vi "KI6221.vi"() -> ()   [LabVIEW 2019] (continued)
  in  "RUN ARB .H":string="The RUN ARB code initiates an ARB waveform. When you see something like \"<PMARK>\" this is a variable. These are replaced with values before being sent to the instrument. Many are self explanatory. DURATION is in seconds and FREQUENCY is in Hz. When you see WAIT1500 that indicates a delay in ms. (i.e. a 1500 ms delay between these commands). When you see ENTER256 this indicates you need to read data from the box. The number is the recommended number of bytes to read. "
  in  "UPLOAD ARB .H":string="The UPLOAD ARB code aborts any other sweep running, turns off the output, then loads an ARB wave. When you see something like \"<PULSELEVEL>\" this is a variable. These are replaced with values before being sent to the instrument. Many are self explanatory. The command sour:wave:arb1:data <WAVEFORM> will upload the waveform to the instrument. The variable needs to be replaced with a sequence of numbers between -1 and 1 separated by commas. I.E. \"1,.5,0,-.5,-1\". The command can only take data about 1000 bytes of ASCII or smaller at a time, so if your waveform is larger than that separate them and use the :sour:wave:arb:append <WAVEFORM> command to add more points. When you see WAIT1500 that indicates a delay in ms. (i.e. a 1500 ms delay between these commands). When you see ENTER256 this indicates you need to read data from the box. The number is the recommended number of bytes to read. "
  in  "RUN PULSE .H":string="The RUN PULSE code aborts any other sweep running, resets the instrument, then sets up a PULSE series. When you see something like \"<PULSELEVEL>\" this is a variable. These are replaced with values before being sent to the instrument. Many are self explanatory. We set the <PULSESWEEPSTATE> to a binary value 1 or 0 depending on whether we want to sweep or repeat pulses. The strings ON and OFF will also work. The <PULSESWEEPINT> variable is used to set the sweep delay. We find that the most repeatable pulses in sweep mode come when you set the delay to 6 ms less than the time that equals the number of NPLCs requested. So the formula for <PULSESWEEPINT> is (NPLC*1/Power_Line_Freq - 6)/1000. The :syst:comm:serial:send command allows communication to the Model 2182 over RS-232. When you see WAIT1500 that indicates a delay in ms. (i.e. a 1500 ms delay between these commands). You may find you have to place additional delays especially when using the RS-232 pass through commands. When you see ENTER256 this indicates you need to read data from the box. The number is the recommended number of bytes to read."
  in  "RUN DC .H":string="The RUN DIFF COND code aborts any other sweep running, resets the instrument, then sets up a DIFF COND sweep. When you see something like \"<DCONSTOP>\" this is a variable. These are replaced with values before being sent to the instrument. Many are self explanatory. We set the DCONSTEP value to (STOP-START)/((NUMPOINTS-1)*FILTERCOUNT) and the DCONDELTA (amplitude of the square wave superimposed on the sweep) is set to STEPSIZE*FILTERCOUNT. The :syst:comm:serial:send command allows communication to the Model 2182 over RS-232. When you see WAIT1500 that indicates a delay in ms. (i.e. a 1500 ms delay between these commands). When you see ENTER256 this indicates you need to read data from the box. The number is the recommended number of bytes to read."
  in  "RUN DELTA .H":string="The RUN DELTA Code aborts any other sweep running, resets the instrument, then sets up a DELTA sweep. When you see something like \"<DELTAHIGH>\" this is a variable. These are replaced with values before being sent to the instrument. Many are self explanatory. The var <DELTACURRRANGE> is the current range and it can be replaced with a numeric string like \" .002\" (2 mA range) or with a string like \":auto on\" which turns auto range on. All other variables will have a space before them. The :syst:comm:serial:send command allows communication to the Model 2182 over RS-232. When you see WAIT1500 that indicates a delay in ms. (i.e. a 1500 ms delay between these commands). When you see ENTER256 this indicates you need to read data from the box. The number is the recommended number of bytes to read."
  out "error out 25":errorcluster
  out "error out 24":errorcluster
  out "error out 23":errorcluster
  out "DELTA SCPI ERROR 2":errorcluster
  out "error out 17":errorcluster
  out "error out 16":errorcluster
  out "Knob Last":i16
  out "Control watch":bool=TRUE
  out "error out 21":errorcluster
  out "error 27":errorcluster
  out "error out 15":errorcluster
  out "SETUP YET?":i32
  out "error out 14":errorcluster
  out "error out 13":errorcluster
  out "VALID SETUP":bool
  out "error out 12":errorcluster
  out "step VISA":refnum<visa-resource-name>="GPIB0::24::INSTR"
  out "6220 VISA":refnum<visa-resource-name>="TCPIP0::10.40.27.160::1394::SOCKET"
  out "GPIB Array":string[](array[string])=["*idn?\nENTER1024", ":SYST:COMM:SERIal:SEND \"*idn?\"\nWAIT1000\n:SYST:COMM:SERIal:enter?\nWAIT1000\nENTER2000", ":disp:data?\nENTER256\n:disp:wind2:data?\nENTER256\n:outp:stat?\nENTER256\n:disp:attr?\nENTER256\n:disp:wind2:attr?\nENTER256", ":syst:key <KEYPRESS>", ":trac:poin:act?\nENTER256", ":sour:wave:arb:append <APPEND>\nWAIT30", "*rst", ":disp:data?\nENTER256\n:disp:wind2:data?\nENTER256\n:outp:stat?\nENTER256\n:disp:attr?\nENTER256\n:disp:wind2:attr?\nENTER256", "sour:swe:abort\nWAIT500\nSOUR:WAVE:ABOR\nWAIT500\noutp:stat off\nsour:wave:ampl <AMPLITUDE>\nsour:wave:offs <OFFSET>\nsour:wave:arb:data <WAVEFORM>\nWAIT300\t", "SOUR:WAVE:ABOR\nWAIT300\n:outp:stat off\n<SETUPSTRING>\nWAIT500\nsour:wave:arb:copy 1\nWAIT3000\nsour:wave:func ARB0\nWAIT1000\nsour:wave:rang best\nsour:wave:pmar:stat <PMARK_ENABLE>\nsour:wave:pmar <PMARK>\nsour:wave:pmar:olin <TRIGGERLINE>\nsour:wave:freq <FREQUENCY>\nsour:wave:dur:time <DURATION>\n:sour:curr:comp <ARBCOMP>\nsour:wave:arm\nWAIT2000\n:outp:stat on\nWAIT500\nsour:wave:init", "SOUR:WAVE:ABOR\noutp:stat off", "sour:wave:arb:poin?\nENTER256", ":sour:delta:nvpr?\nENTER256", ":sour:dcon:nvpr?\nENTER256", ":SYST:COMM:SERIal:SEND \"*rst\"\nWAIT1500\n:sour:pdel:nvpr?\nENTER256", "SOUR:WAVE:ABOR\noutp:stat off\n*rst", ":sour:swe:abort\n*rst\n<SETUPSTRING>\nWAIT500\n:form:elem READ,TST,RNUM,AVOL\n:sour:delt:high <DELTAHIGH>\n:sour:delt:low <DELTALOW>\n:sour:delt:count <DELTANUMCYCLE>\n:sour:delt:delay <DELTADELAY>\n:sour:curr:filt:stat <DELTADAMPING>\n:sour:curr:comp <DELTACOMP>\n:sour:curr:rang<DELTACURRRANGE>\n:SYST:COMM:SERIal:SEND \"*rst\"\nWAIT400\n:SYST:COMM:SERIal:SEND \":sens:volt:nplc <DELTANPLC>\"\nWAIT1500\n:SYST:COMM:SERIal:SEND \":sens:volt:rang <DELTAVOLTRANGE>\"\n:sens:aver:wind 0\n:sens:aver:stat <DELTAFILTERSTATE>\n:sens:aver:coun <DELTAFILTERCOUNT>\n:sens:aver:tcon <DELTAFILTERTYPE>\n:sour:delt:arm\nWAIT1000\n:init:imm", ":sour:swe:abort\n:outp:stat off", ":sour:swe:abort\n:outp:stat off", ":trac:data:sel? <DATASTART>,<DATACOUNT>\nENTER40000", ":sour:swe:abort\nWAIT3000\n*rst\n<SETUPSTRING>\nWAIT500\n:form:elem READ,TST,RNUM,SOUR\n:sour:pdel:high <PULSEHIGH>\n:sour:pdel:low <PULSEOFF>\n:sour:pdel:count <PULSECOUNT>\n:sour:pdel:rang best\n:sour:swe:rang best\n:sour:pdel:width <PULSEWIDTH>\n:sour:pdel:sdel <PULSEDELAY>\n:sour:pdel:swe <PULSESWEEPSTATE>\n:sour:pdel:int <PULSEINTERVAL>\n:sour:curr:comp <PULSECOMP>\n:sour:swe:spac <PULSESWEEPSPACING>\n:sour:curr:start <PULSESWEEPSTART>\n:sour:curr:stop <PULSESWEEPSTOP>\n:sour:curr:step <PULSESWEEPSTEP>\n:SYST:COMM:SERIal:SEND \":sens:volt:rang <PULSEVOLTRANGE>\"\n:sens:aver:wind 0\n:sens:aver:stat <PULSEFILTERSTATE>\n:sens:aver:coun <PULSEFILTERCOUNT>\n:sens:aver:tcon <PULSEFILTERTYPE>\n:sour:pdel:arm\nWAIT3000\n:init:imm", ":sour:swe:abort\n:outp:stat off", ":sour:swe:abort", ":trac:data:sel? 0,<DATACOUNT>\nENTER4000000", ":sour:swe:abort\n*rst\n<SETUPSTRING>\nWAIT500\n:form:elem READ,TST,RNUM,SOUR,AVOL\n:sour:dcon:start <DCONSTART>\n:sour:dcon:stop <DCONSTOP>\n:sour:dcon:step <DCONSTEP>\n:sour:dcon:del <DCONDELAY>\n:sour:dcon:delt <DCONDELTA>\n:sour:curr:comp <DCONCOMP>\n:sour:curr:filt:stat <DCONDAMPING>\n:SYST:COMM:SERIal:SEND \":sens:volt:rang <DCONVOLTRANGE>\"\nWAIT700\n:SYST:COMM:SERIal:SEND \":sens:volt:nplc <DCONNPLC>\"\nWAIT500\n:sens:aver:wind 0\n:sens:aver:stat <DCONFILTERSTATE>\n:sens:aver:coun <DCONFILTERCOUNT>\n:sens:aver:tcon REPEAT\nWAIT2000\n:sour:dcon:arm\nWAIT3000\n:init:imm", ":sour:swe:abort\n:outp:stat off", ":sour:swe:abort", ":sour:swe:abort\nWAIT2000\n:outp:stat off\n*rst\nWAIT1000\n:sour:curr:comp <AUTOCOMP>\n:sour:curr:filt:stat <DCONDAMPING>\n:SYST:COMM:SERIal:SEND \"*rst\"\nWAIT800\n:SYST:COMM:SERIal:SEND \":sens:volt:rang <DCONVOLTRANGE>\"\nWAIT200\n:SYST:COMM:SERIal:SEND \":sens:volt:rang:auto on\"\nWAIT200\n:SYST:COMM:SERIal:SEND \":sens:volt:nplc <DCONNPLC>\"\nWAIT200", ":sour:curr:rang <STARTLEVEL>\n:sour:curr:lev <STARTLEVEL>\n:outp:stat on\nWAIT200\n:sour:curr:rang <CURRENTLEVEL>\n:sour:curr:lev <CURRENTLEVEL>\nWAIT500\n:SYST:COMM:SERIal:SEND \":read?\"\nWAIT1000\n:SYST:COMM:SERIal:enter?\nENTER512", ":sour:curr:rang <SOURCE>\n:sour:curr:lev <SOURCE>\n:sour:curr:comp <COMPLIANCE>\n:outp:stat <OUTPUT>", ":sour:swe:abort\n*rst\n<SETUPSTRING>\nWAIT1000\n:sour:swe:spac <SPACING>\n:sour:swe:poin <POINTS>\n:sour:swe:rang best\n:sour:swe:coun 1\n:sour:swe:cab off\n:sour:curr:start <STARTLEVEL>\n:sour:curr:stop <STOPLEVEL>\n:sour:curr:comp <COMPLIANCE>\n:sour:del <DELAY>\nWAIT1000\n:sour:swe:arm\nWAIT3000\n:init:imm", ":sour:swe:abort\n:outp:stat off", "#33 basic AC Source STOP%", "#34 wAIT%\nWAIT2000", "WAIT2000", ":sour:swe:abort\n*rst\n:SYST:COMM:SERIal:SEND \"*rst\"\n<SETUPSTRING>\nWAIT1000\n:sour:swe:spac <SPACING>\n:sour:swe:poin <POINTS>\n:sour:swe:rang best\n:sour:swe:coun 1\n:sour:swe:cab off\n:sour:curr:start <STARTLEVEL>\n:sour:curr:stop <STOPLEVEL>\n:sour:curr:comp <COMPLIANCE>\n:sour:del <DELAY>\n:trig:sour tlink\n:trig:dir sour\n:trig:olin 2\n:trig:ilin 1\n:trig:outp del\n:SYST:COMM:SERIal:SEND \":sens:volt:rang <VOLTRANGE>\"\nWAIT400\n:SYST:COMM:SERIal:SEND \":sens:volt:nplc <NPLC>\"\nWAIT400\n:SYST:COMM:SERIal:SEND \":trac:cle\"\nWAIT200\n:SYST:COMM:SERIal:SEND \":trac:feed sens\"\nWAIT200\n:SYST:COMM:SERIal:SEND \":trac:poin <POINTS>\"\nWAIT200\n:SYST:COMM:SERIal:SEND \":trig:sour ext\"\nWAIT200\n:SYST:COMM:SERIal:SEND \":trig:coun <POINTS>\"\nWAIT200\n:SYST:COMM:SERIal:SEND \":trac:feed:control next\"\nWAIT500\n:sour:swe:arm\nWAIT1000\n:init:imm\n:SYST:COMM:SERIal:SEND \"init\"", ":sour:swe:abort\n:outp:stat off\n*rst\n:SYST:COMM:SERIal:SEND \"*rst\"\n:trig:olin 4", "*idn?\nENTER1024\n:sour:swe:abort\n*rst\n<SETUPSTRING>\nWAIT1000", ":SYST:COMM:SERIal:SEND \":trac:data?\"\nWAIT200\n:SYST:COMM:SERIal:enter?\nENTER40000", ":sour:wave:abor\nWAIT300\n:outp:stat off\n*rst\nWAIT2000\n<SETUPSTRING>\n:sour:curr:comp <ACCOMPLIANCE>\n:sour:wave:func ramp\n:sour:wave:rang best\n:sour:wave:dcycle <RAMPDUTYCYCLE>\n:sour:wave:ampl <RAMPAMPLITUDE>\n:sour:wave:freq <FREQUENCY>\n:sour:wave:offset <RAMPOFFSET>\n:sour:wave:dur:time inf\n:sour:wave:arm\nWAIT3000\n:sour:wave:init", ":sour:wave:abor\nWAIT300\n:outp:stat off\n*rst\nWAIT2000\n<SETUPSTRING>\nWAIT500\n:sour:curr:comp <ACCOMPLIANCE>\n:sour:wave:func square\n:sour:wave:dcycle <SQUAREDUTYCYCLE>\n:sour:wave:ampl <SQUAREAMPLITUDE>\n:sour:wave:freq <FREQUENCY>\n:sour:wave:offset <SQUAREOFFSET>\n:sour:wave:rang best\n:sour:wave:dur:time inf\n:sour:wave:arm\nWAIT3000\n:sour:wave:init", ":sour:wave:abor\nWAIT300\n:outp:stat off\n*rst\nWAIT2000\n<SETUPSTRING>\nWAIT500\n:sour:curr:comp <ACCOMPLIANCE>\n:sour:wave:func sin\n:sour:wave:ampl <SINEAMPLITUDE>\t\t\n:sour:wave:freq <FREQUENCY>\n:sour:wave:offset <SINEOFFSET>\n:sour:wave:rang best\n:sour:wave:dur:time inf\n:sour:wave:arm\nWAIT3000\n:sour:wave:init", ""]
  out "error out 10":errorcluster
  out "error out 7":errorcluster
  out "triggerline":i16=1 min=0 max=5
  out "Phase Value":dbl min=0.0 max=360.0
  out "phase enable":bool
  out "error out 5":errorcluster
  out "selection":dbl[](array[numeric])=[2.01, 2.01, 2.01, 2.01, 2.01, 1.99, 1.99, 1.99, 1.99, 1.99, 2.01, 2.01, 2.01, 2.01, 2.01, 1.99, 1.99, 1.99, 1.99, 1.99, 2.01, 2.01, 2.01, 2.01, 2.01, 1.99, 1.99, 1.99, 1.99, 1.99, 2.01, 2.01, 2.01, 2.01, 2.01, 1.99, 1.99, 1.99, 1.99, 1.99, 2.01, 2.01, 2.01, 2.01, 2.01, 1.99, 1.99, 1.99, 1.99, 1.99, 2.01, 2.01, 2.01, 2.01, 2.01, 1.99, 1.99, 1.99, 1.99, 1.99, 2.01, 2.01, 2.01, 2.01, 2.01, 1.99, 1.99, 1.99, 1.99, 1.99, 2.01, 2.01, 2.01, 2.01, 2.01, 1.99, 1.99, 1.99, 1.99, 1.99, 2.01, 2.01, 2.01, 2.01, 2.01, 1.99, 1.99, 1.99, 1.99, 1.99, 2.01, 2.01, 2.01, 2.01, 2.01, 1.99, 1.99, 1.99, 1.99, 1.99]
  out "Pad Last":i32=-2
  out "Graph Last":i32=-2
  in  "waveform holder":dbl[](array[numeric])
  out "empty":dbl[](array[numeric])
  out "Complete Array Cnt":i32[](array[numeric])
  out "ScratchPad Array Cnt":i32[](array[numeric])=[100, 100, 100, 100, 0]
  out "Default path":path=path "C:/6220software/data"
  out "error out 6":errorcluster
  out "Complete Array":dbl[][](array[numeric])
  out "ScratchPad Array":dbl[][](array[numeric])
  in  "mail server":string
  in  "attachments":T6(array[cluster])=[{"path"=path "C:/6220software/data/DefaultTestFile.cfg", "data"="", "binary"=FALSE, "MIME content-type \n(application/octet-stream)"=""}, {"path"=path "C:/6220software/data/DefaultTestFile_dcdata.cfg", "data"="", "binary"=FALSE, "MIME content-type \n(application/octet-stream)"=""}, {"path"=path "C:/6220software/data/DefaultTestFile_pulsedata.cfg", "data"="", "binary"=FALSE, "MIME content-type \n(application/octet-stream)"=""}, {"path"=path "C:/6220software/data/DefaultTestFile_deltadata.cfg", "data"="", "binary"=FALSE, "MIME content-type \n(application/octet-stream)"=""}]
  out "error out 4":errorcluster
  out "Y AXIS LAST -PULSE":i32=-1
  in  "Y AXIS LAST -DC":i32=-1
  out "Y AXIS LAST -DELTA":i32
  out "X AXIS LAST -PULSE":i32
  in  "X AXIS LAST -DC":i32
  out "X AXIS LAST -DELTA":i32
  out "DELTA SCPI ERROR":errorcluster
  out "Settings cluster":T7={"Boolean"=TRUE, "Numeric"=5.0, "y"=timestamp(3168632206.8599997 s since 1904-01-01), "version"="2.6", "y 2"=timestamp(3168632206.8599997 s since 1904-01-01)}
  out "FIRST OPEN":bool
  out "Last setup Cluster":T8={"Numeric"=2, "Numeric 2"=3, "Numeric 3"=1, "Numeric 4"=10, "Numeric 5"=40, "Numeric 6"=27, "Numeric 7"=160, "Numeric 8"=0, "Numeric 9"=16, "Numeric 10"=0, "Numeric 11"=1, "Numeric 12"=0, "Numeric 13"=0, "Boolean"=FALSE, "Numeric 14"=0, "Numeric 15"=0}
  out "error out 2":errorcluster
  in  "Default Cluster":T8={"Numeric"=2, "Numeric 2"=3, "Numeric 3"=1, "Numeric 4"=10, "Numeric 5"=40, "Numeric 6"=27, "Numeric 7"=160, "Numeric 8"=0, "Numeric 9"=16, "Numeric 10"=0, "Numeric 11"=1, "Numeric 12"=0, "Numeric 13"=0, "Boolean"=FALSE, "Numeric 14"=0, "Numeric 15"=0}
  out "MASTER DRIVER Array":T9(array[cluster])=[{"Numeric"=24, "String"="2400", "String 2"="*IDN?", "String 3"="2400", "String 4"="*rst\n:sour:func volt\n:outp:stat on", "String 5"=":sour:volt:lev <LEVEL>", "String 6"=":outp:stat off", "Numeric 2"=20}, {"Numeric"=20, "String"="Window Pop-up", "String 2"="", "String 3"="", "String 4"="THIS IS A SPECIAL SETUP FUNCTION THAT CREATES A POP-UP WINDOW SO YOU CAN SET SOME MANUAL EXTERNAL DEVICE TO THE APPROPRIATE STEP VALUES.\nDO NOT EDIT THIS SETUP OR CHANGE THE INSTRUMENT NAME.", "String 5"="", "String 6"="", "Numeric 2"=20}, {"Numeric"=20, "String"="NEW...", "String 2"="", "String 3"="", "String 4"="", "String 5"="", "String 6"="", "Numeric 2"=20}]
  out "STEP EDIT VAR":bool
  out "output cluster":T10={"Value"=0.0004, "Value"=50, "Value"=1, "Value"=FALSE, "Value"=-0.0004, "Value"=1000, "Value"=0, "Value"=1.0, "Value"=0.01, "Value"=FALSE, "Value"=1.0, "Value"=10.0, "Value"=0, "Value"=0.0, "Value"=-0.001, "Value"=101, "Value"=0.0, "Value"=0.001, "Value"=2, "Value"=101, "Value"=1, "Value"=0, "Value"=2.0, "Value"=0.0, "Value"=1, "Value"=FALSE, "Value"=1.0, "Value"=100, "Value"=2, "Value"=2, "Value"=0.01, "Value"=0.0, "Value"=0, "Value"=10.0, "Value"=1.0, "Value"=100.0, "Value"=0.1, "Value"=0, "Value"=10000.0, "Value"=100, "complete number of cycles"=10.0, "Value"=20, "Value"=0.016, "Value"=0.05, "Value"=0.01, "Value"=0.01, "Value"=0.0, "Value"=0, "Value"=0.05, "Value"=100.0, "Value"=10.0, "Value"=0, "Value"=1, "Value"=FALSE, "Value"=40, "Value"=3, "Value"=0, "Value"=FALSE, "Value"=1, "Value"=10, "Value"=0, "Value"=0, "Value"=1, "Value"=27, "Value"=TRUE, "Value"=2, "Value"=160, "Value"=16, "Value"=TRUE, "Value"=0, "result string"="2400", "result string"="*rst\n:sour:func volt\n:outp:stat on", "result string"=":outp:stat off", "result string"=":sour:volt:lev <LEVEL>", "result string"="*IDN?", "result string"="2400", "Value"=20, "Value"=24, "Value"=FALSE, "String"="Enter details to remember about this test here. It will be saved with your test file.", "PULSE - SWEEP #STEPS"=101, "Sawtooth NUM CYCLES"=5.0, "Sawtooth Offset (Amps) 2"=0.01, "Duty Cycle (%) 2"=50.0, "Start Phase \n(Degrees) 2"=0.0, "SQUARE Number of Points per cycle 2"=10, "SQUARE Number of Cycles 2"=10.0, "SQUARE Amplitude (Amps) 2"=0.01, "SQUARE Offset (Amps) 2"=0.0, "SQUARE Duty Cycle (%) 3"=50.0, "SQUARE Start Phase \n(Degrees) 3"=0.0, "SQUARE Rise/Fall in points 2"=1, "SINE Number of Points per cycle 2"=100, "SINE Number of Cycles 2"=1.0, "SINE Amplitude (Amps) 2"=0.05000000000000075, "SINE Offset (Amps) 2"=0.0, "SINE Start Phase \n(Degrees) 3"=0.0, "NOISE Number of Points per cycle 2"=100, "NOISE Number of Cycles 2"=1.0, "NOISE Standard Deviation 2"=0.01, "NOISE Offset (Amps) 2"=0.0, "Analog filter - \nTau in # points 2"=1.0, "ScratchPad Array 2"=array4x66001[264004 elements], "ScratchPad Array Cnt 2"=[100, 100, 100, 100, 0], "Item Names"=["RAMP0", "SQUARE0", "SINE0", "NOISE0"], "ADD 5"=[2], "Complete Array 2"=[], "Complete Array Cnt 2"=[0], "Item Names 5"=[], "ADD 7"=[0], "waveform holder 2"=[], "ADD 6"=[1], "ADD 8"=[1], "ADD 9"=[1], "Trace offset (% Pk-Pk): 2"=0.0, "phase enable 2"=FALSE, "Phase Value 2"=0.0, "triggerline 2"=1, "Pulse Off Level (Amps) 2"=0.0, "ARB VOLT COMP"=10.0, "nV CAP"=0, "Pulse Filter"=0, "Pulse FIlter Count"=2, "Setup String"=":SYST:COMM:SERIal:SEND \"SYST:FFIL ON\"\r\n:OUTP:ISH OLOW\r\n:outp:lte OFF", "DCON filter state"=0, "Source Level (Amps) 3"=0.0, "Current Source \nVoltage Compliance (V) 4"=10.01, "Start Current (Amps) 3"=0.001, "Stop Current (Amps) 3"=0.005, "Number of sweep points 3"=50, "Sweep Type 3"=0, "Current Source \nVoltage Compliance (V) 5"=10.0, "Delay (settle time in sec) 3"=0.01, "enable measure 3"=TRUE, "Voltage Measure Range 3"=0.1, "Measurement Integration \n(NPLCs) 3"=1.0, "Waveform Type  3"=1, "I Sweep V Measure Data 3"=[], "Ramp from: (Amps) 3"=0.0, "Ramp to: (Amps) 3"=0.0, "Duty Cycle (%) 4"=50.0, "Amplitude (Amps) 4"=0.105, "Offset (Amps) 4"=0.0, "Duty Cycle (%) 5"=50.0, "Amplitude (Amps) 5"=2e-12, "Offset (Amps) 5"=0.01, "Signal Repetition \nFrequency (Hz) 3"=10.0, " Voltage\n Compliance3"=10.0, "Number of Zero Measurements 2"=0} {"Number of Zero Measurements 2" min=0 max=2 step=1; "Voltage\n Compliance3" min=0.1 max=105.0 step=0.01 format="%#_3f"; "Signal Repetition \nFrequency (Hz) 3" min=0.0001 max=100000.0 format="%.4f"; "Offset (Amps) 5" min=-0.105 max=0.105 step=1e-12 format="%^#.6g"; "Amplitude (Amps) 5" min=2e-12 max=0.105 step=1e-12 format="%^#_6g"; "Duty Cycle (%) 5" min=0.0 max=100.0 format="%#.2f"; "Offset (Amps) 4" min=-0.105 max=0.105 step=1e-12 format="%^#_6g"; "Amplitude (Amps) 4" min=0.0 max=0.105 step=1e-12 format="%^#.6g"; "Duty Cycle (%) 4" min=0.0 max=100.0 format="%#.2f"; "Ramp to: (Amps) 3" min=-0.105 max=0.105 step=1e-12 format="%^#_6g"; "Ramp from: (Amps) 3" min=-0.105 max=0.105 step=1e-12 format="%^#.6g"; "Waveform Type  3" items=["RAMP", "SQUARE", "SINE"]; "Measurement Integration \n(NPLCs) 3" items=["0.01"=0.01, "0.1"=0.1, "1"=1.0, "10"=10.0]; "Voltage Measure Range 3" items=["10 mV"=0.01, "100 mV"=0.1, "1 V"=1.0, "10 V"=10.0, "100 V"=100.0]; "Delay (settle time in sec) 3" min=0.001 max=9999000.0 format="%^#_6g"; "Current Source \nVoltage Compliance (V) 5" min=0.1 max=105.0 step=0.01 format="%^#_6g"; "Sweep Type 3" items=["Linear ", "Logarithmic"]; "Number of sweep points 3" min=2 max=65536; "Stop Current (Amps) 3" min=-0.105 max=0.105 format="%^#_6g"; "Start Current (Amps) 3" min=-0.105 max=0.105 format="%^#_6g"; "Current Source \nVoltage Compliance (V) 4" min=0.1 max=105.0 step=0.01 format="%^#_6g"; "Source Level (Amps) 3" min=-0.105 max=0.105 step=1e-12 format="%^#_9e"; "Pulse Off Level (Amps) 2" min=-0.1 max=0.1 format="%^#_3e"; "triggerline 2" min=0 max=5; "Phase Value 2" min=0.0 max=360.0; "Analog filter - \nTau in # points 2" min=1.0; "NOISE Offset (Amps) 2" min=-10.0 max=10.0 format="%^#_6e"; "NOISE Standard Deviation 2" min=0.0 max=1.0 format="%^#_6e"; "NOISE Number of Cycles 2" min=1.0 max=65536.0; "NOISE Number of Points per cycle 2" min=1 max=65536 format="%#.0f"; "SINE Start Phase \n(Degrees) 3" min=0.0 max=360.0 format="%#.3f"; "SINE Offset (Amps) 2" min=-10.0 max=10.0 step=1e-17 format="%#.2f"; "SINE Amplitude (Amps) 2" min=-10.0 max=10.0 step=1e-12 format="%^#_6e"; "SINE Number of Cycles 2" min=1.0 max=65536.0; "SINE Number of Points per cycle 2" min=1 max=65536 format="%#.0f"; "SQUARE Rise/Fall in points 2" min=1; "SQUARE Start Phase \n(Degrees) 3" min=0.0 max=360.0 format="%#.3f"; "SQUARE Duty Cycle (%) 3" min=0.0 max=100.0 format="%#.2f"; "SQUARE Offset (Amps) 2" min=-10.0 max=10.0 format="%^#_6e"; "SQUARE Amplitude (Amps) 2" min=-10.0 max=10.0 format="%^#.6e"; "SQUARE Number of Cycles 2" min=1.0; "SQUARE Number of Points per cycle 2" min=1; "Start Phase \n(Degrees) 2" min=0.0 max=360.0 format="%#.3f"; "Duty Cycle (%) 2" min=0.0 max=100.0 format="%#.2f"; "Sawtooth Offset (Amps) 2" min=-10.0 max=10.0 format="%^#_6e"; "Sawtooth NUM CYCLES" min=1.0}
  out "SAVE NOW":bool
  out "EXIT NOW":bool
  # "Model 6220/6221 Current Source Example Software"
  # "Instrument Communication"
  # "Last Saved settings open on startup..."
  # "Instrument Selection"
  # "Source Connection"
  # "Measure Connection"
  # "Communication Configuration"
  # "Earth Connection"
  # "Input Capacitance"
  # "Step-By-Step Instrument Connection Tutorial"
  # "Connect communication cables as shown:"
  # "Connect the current source to the DUT as shown:"
  # "Connect the nanovoltmeter to the DUT as shown:"
  # "Select problems to view best shielding configuration:"
  # "Data Sheet"
  # "Data Sheet"
  # "Horizontal and Vertical Axis are controlled from 2-D Graph Tab"
  # "Data Sheet"
  # "Z data controlled by step source values:"
  # "For one sweep, set # of steps to 1 and set the Start Level."
  # "Data Sheet"
  # "Waveforms     ----------->               ScratchPad                 ------>                Complete waveform settings"
  # "Browse to a file containing your points. File should be\na text file with CRLFs between each point. This is the\ntype of waveform where you can customize a wave\nin a spreadsheet editor or other tool. Simply, create a\nsingle column of data points in column A on a blank\nsheet and select to save the sheet as a text file. This\nshould work by default, but it can be checked by \nopening with Notepad. Data should appear as a \ncolumn of text with carriage returns after each point."
  # "Select the waves you wish to combine in a calculation\nor check the box next to Constant and use the left \nselection and constant in scalar math.\nThen click CREATE."
  # "Select a waveform from the scratchpad to apply an\nanalog filter. Then click CREATE."
  # "6220 Virtual Instrument Front Panel"
  # "First, click Take Control of Instrument. Then use buttons and knobs below as you would from the instrument front panel. \nConnection uses settings on Instrument Communication Panel."
  # "Go Online..."
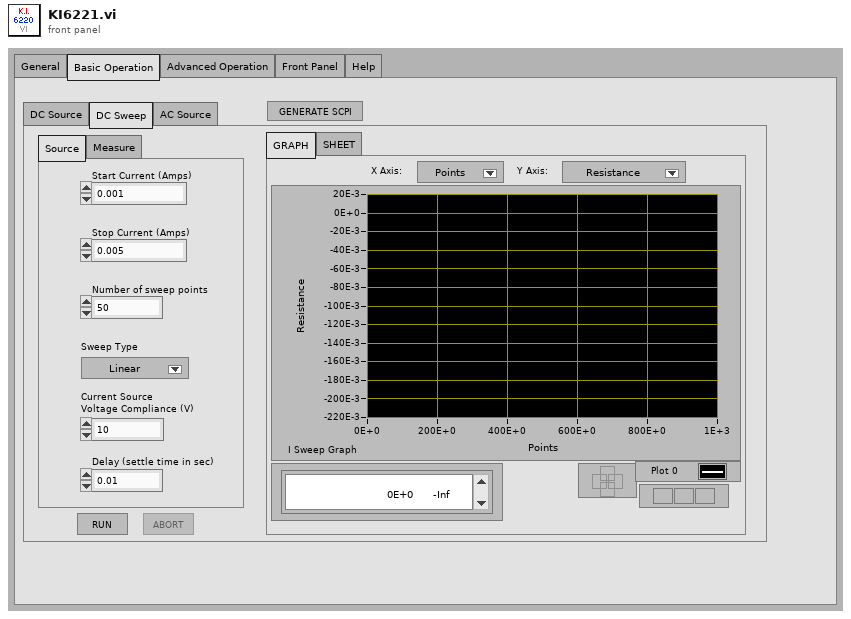
[diagram p1: front panel]
types:
  T1 = enum32{"General", "Basic Operation", "Advanced Operation", "Front Panel", "Help"}
  T2 = enum32{"STARTUP", "CONN CONFIG", "CONN GUIDE", "STEP CONFIG"}
  T3 = enum32{"step 1", "step 2", "step 3", "step 4", "final"}
  T4 = enum32{"Delta Mode Measurements", "Differential Conductance Measurements", "Pulsed IV Measurements", "ARB Waveform Generator", "6220 Virtual Front Panel", "Instrument Communication"}
  T5 = enum32{"RAMP", "SQUARE", "SINE", "NOISE", "CUSTOM", "CALCULATED", "FILTER"}
  T6 = cluster{"path":path, "data":string, "binary":bool, "MIME content-type \n(application/octet-stream)":string}[]
  T7 = cluster{"Boolean":bool, "Numeric":dbl, "y":timestamp, "version":string, "y 2":timestamp}
  T8 = cluster{"Numeric":i32, "Numeric 2":i32, "Numeric 3":i32, "Numeric 4":i32, "Numeric 5":i32, "Numeric 6":i32, "Numeric 7":i32, "Numeric 8":i32, "Numeric 9":i32, "Numeric 10":i32, "Numeric 11":i32, "Numeric 12":i32, "Numeric 13":i32, "Boolean":bool, "Numeric 14":u16, "Numeric 15":u16}
  T9 = cluster{"Numeric":i32, "String":string, "String 2":string, "String 3":string, "String 4":string, "String 5":string, "String 6":string, "Numeric 2":i32}[]
  T10 = cluster{"Value":dbl, "Value":i32, "Value":u16, "Value":bool, "Value":dbl, "Value":i32, "Value":u16, "Value":dbl, "Value":dbl, "Value":bool, "Value":dbl, "Value":dbl, "Value":u16, "Value":dbl, "Value":dbl, "Value":i32, "Value":dbl, "Value":dbl, "Value":u16, "Value":i32, "Value":u16, "Value":u16, "Value":dbl, "Value":dbl, "Value":u16, "Value":bool, "Value":dbl, "Value":i32, "Value":i32, "Value":u16, "Value":dbl, "Value":dbl, "Value":u16, "Value":dbl, "Value":dbl, "Value":dbl, "Value":dbl, "Value":u16, "Value":dbl, "Value":i32, "complete number of cycles":dbl, "Value":i32, "Value":dbl, "Value":dbl, "Value":dbl, "Value":dbl, "Value":dbl, "Value":u16, "Value":dbl, "Value":dbl, "Value":dbl, "Value":u16, "Value":u16, "Value":bool, "Value":i32, "Value":u16, "Value":i32, "Value":bool, "Value":u16, "Value":i32, "Value":u16, "Value":u16, "Value":u16, "Value":i32, "Value":bool, "Value":u16, "Value":i32, "Value":i32, "Value":bool, "Value":i32, "result string":string, "result string":string, "result string":string, "result string":string, "result string":string, "result string":string, "Value":i32, "Value":i32, "Value":bool, "String":string, "PULSE - SWEEP #STEPS":i32, "Sawtooth NUM CYCLES":dbl, "Sawtooth Offset (Amps) 2":dbl, "Duty Cycle (%) 2":dbl, "Start Phase \n(Degrees) 2":dbl, "SQUARE Number of Points per cycle 2":i32, "SQUARE Number of Cycles 2":dbl, "SQUARE Amplitude (Amps) 2":dbl, "SQUARE Offset (Amps) 2":dbl, "SQUARE Duty Cycle (%) 3":dbl, "SQUARE Start Phase \n(Degrees) 3":dbl, "SQUARE Rise/Fall in points 2":i32, "SINE Number of Points per cycle 2":i32, "SINE Number of Cycles 2":dbl, "SINE Amplitude (Amps) 2":dbl, "SINE Offset (Amps) 2":dbl, "SINE Start Phase \n(Degrees) 3":dbl, "NOISE Number of Points per cycle 2":i32, "NOISE Number of Cycles 2":dbl, "NOISE Standard Deviation 2":dbl, "NOISE Offset (Amps) 2":dbl, "Analog filter - \nTau in # points 2":dbl, "ScratchPad Array 2":dbl[][], "ScratchPad Array Cnt 2":i32[], "Item Names":string[], "ADD 5":i32[], "Complete Array 2":dbl[][], "Complete Array Cnt 2":i32[], "Item Names 5":string[], "ADD 7":i32[], "waveform holder 2":dbl[], "ADD 6":i32[], "ADD 8":i32[], "ADD 9":i32[], "Trace offset (% Pk-Pk): 2":dbl, "phase enable 2":bool, "Phase Value 2":dbl, "triggerline 2":i16, "Pulse Off Level (Amps) 2":dbl, "ARB VOLT COMP":dbl, "nV CAP":u16, "Pulse Filter":u16, "Pulse FIlter Count":i32, "Setup String":string, "DCON filter state":u16, "Source Level (Amps) 3":dbl, "Current Source \nVoltage Compliance (V) 4":dbl, "Start Current (Amps) 3":dbl, "Stop Current (Amps) 3":dbl, "Number of sweep points 3":i32, "Sweep Type 3":u16, "Current Source \nVoltage Compliance (V) 5":dbl, "Delay (settle time in sec) 3":dbl, "enable measure 3":bool, "Voltage Measure Range 3":dbl, "Measurement Integration \n(NPLCs) 3":dbl, "Waveform Type  3":u16, "I Sweep V Measure Data 3":string[][], "Ramp from: (Amps) 3":dbl, "Ramp to: (Amps) 3":dbl, "Duty Cycle (%) 4":dbl, "Amplitude (Amps) 4":dbl, "Offset (Amps) 4":dbl, "Duty Cycle (%) 5":dbl, "Amplitude (Amps) 5":dbl, "Offset (Amps) 5":dbl, "Signal Repetition \nFrequency (Hz) 3":dbl, " Voltage\n Compliance3":dbl, "Number of Zero Measurements 2":i32}
  T11 = cluster{"Numeric":i32, "Numeric 2":i32, "Numeric 3":i32, "Numeric 4":i32, "Numeric 5":i32, "Numeric 6":i32, "Numeric 7":i32, "Numeric 8":i32, "Numeric 9":i32, "Numeric 10":i32, "Numeric 11":i32, "Numeric 12":i32, "Numeric 13":i32, "Boolean":bool, "Numeric 16":u16, "Numeric 17":u16}
  T12 = typedef "LVRectTypeDef.ctl" = cluster{"Left":i16, "Top":i16, "Right":i16, "Bottom":i16}
  T13 = typedef "imagedata.ctl" = cluster{"image type":i32, "image depth":i32, "image":u8[], "mask":u8[], "colors":u32[], "Rectangle":cluster{"left":i16, "top":i16, "right":i16, "bottom":i16}}
  T14 = cluster{"Numeric":i32, "String":string, "String 2":string, "String 3":string, "String 4":string, "String 5":string, "String 6":string, "Numeric 2":i32}
  T15 = cluster{"Value":dbl, "Value":i32, "Value":u16, "Value":bool, "Value":dbl, "Value":i32, "Value":u16, "Value":dbl, "Value":dbl, "Value":bool, "Value":dbl, "Value":dbl, "Value":u16, "Value":dbl, "Value":dbl, "Value":i32, "Value":dbl, "Value":dbl, "Value":u16, "Value":i32, "Value":u16, "Value":u16, "Value":dbl, "Value":dbl, "Value":u16, "Value":bool, "Value":dbl, "Value":i32, "Value":i32, "Value":u16, "Value":dbl, "Value":dbl, "Value":u16, "Value":dbl, "Value":dbl, "Value":dbl, "Value":dbl, "Value":u16, "Value":dbl, "Value":i32, "complete number of cycles":dbl, "Value":i32, "Value":dbl, "Value":dbl, "Value":dbl, "Value":dbl, "Value":dbl, "Value":u16, "Value":dbl, "Value":dbl, "Value":dbl, "Value":u16, "Value":u16, "Value":bool, "Value":i32, "Value":u16, "Value":i32, "Value":bool, "Value":u16, "Value":i32, "Value":u16, "Value":u16, "Value":u16, "Value":i32, "Value":bool, "Value":u16, "Value":i32, "Value":i32, "Value":bool, "Value":i32, "result string":string, "result string":string, "result string":string, "result string":string, "result string":string, "result string":string, "Value":i32, "Value":i32, "Value":bool, "String":string, "PULSE - SWEEP #STEPS":i32, "Sawtooth NUM CYCLES":dbl, "Sawtooth Offset (Amps) 2":dbl, "Duty Cycle (%) 2":dbl, "Start Phase \n(Degrees) 2":dbl, "SQUARE Number of Points per cycle 2":i32, "SQUARE Number of Cycles 2":dbl, "SQUARE Amplitude (Amps) 2":dbl, "SQUARE Offset (Amps) 2":dbl, "SQUARE Duty Cycle (%) 3":dbl, "SQUARE Start Phase \n(Degrees) 3":dbl, "SQUARE Rise/Fall in points 2":i32, "SINE Number of Points per cycle 2":i32, "SINE Number of Cycles 2":dbl, "SINE Amplitude (Amps) 2":dbl, "SINE Offset (Amps) 2":dbl, "SINE Start Phase \n(Degrees) 3":dbl, "NOISE Number of Points per cycle 2":i32, "NOISE Number of Cycles 2":dbl, "NOISE Standard Deviation 2":dbl, "NOISE Offset (Amps) 2":dbl, "Analog filter - \nTau in # points 2":dbl, "ScratchPad Array 2":dbl[][], "ScratchPad Array Cnt 2":i32[], "Item Names":string[], "ADD 5":i32[], "Complete Array 2":dbl[][], "Complete Array Cnt 2":i32[], "Item Names 5":string[], "ADD 7":i32[], "waveform holder 2":dbl[], "ADD 6":i32[], "ADD 8":i32[], "ADD 9":i32[], "Trace offset (% Pk-Pk): 2":dbl, "phase enable 2":bool, "Phase Value 2":dbl, "triggerline 2":i16, "Pulse Off Level (Amps) 2":dbl, "ARB VOLT COMP":dbl, "nV CAP":u16, "Pulse Filter 2":u16, "Pulse FIlter Count 2":i32, "Setup String":string, "DCON filter state":u16, "Source Level (Amps) 3":dbl, "Current Source \nVoltage Compliance (V) 4":dbl, "Start Current (Amps) 3":dbl, "Stop Current (Amps) 3":dbl, "Number of sweep points 3":i32, "Sweep Type 3":u16, "Current Source \nVoltage Compliance (V) 5":dbl, "Delay (settle time in sec) 3":dbl, "enable measure 3":bool, "Voltage Measure Range 3":dbl, "Measurement Integration \n(NPLCs) 3":dbl, "Waveform Type  3":u16, "I Sweep V Measure Data 3":string[][], "Ramp from: (Amps) 3":dbl, "Ramp to: (Amps) 3":dbl, "Duty Cycle (%) 4":dbl, "Amplitude (Amps) 4":dbl, "Offset (Amps) 4":dbl, "Duty Cycle (%) 5":dbl, "Amplitude (Amps) 5":dbl, "Offset (Amps) 5":dbl, "Signal Repetition \nFrequency (Hz) 3":dbl, " Voltage\n Compliance3":dbl, "Number of Zero Measurements 2":i32}
diagram:
  # "CLOSE THE FRONT PANEL"
  # "ENTER WHILE LOOP. THIS IS THE MAIN PROGRAM EXECUTION ENGINE. ONLY EXIT WHILE LOOP ON EXIT BUTTON AFTER SAVE PROMPT.\nMAIN CASE IS THE MAIN TABS SET...BUTTONS ACROSS TOP OF FRONT PANEL ARE ATTACHED TO CASE STATEMENTS TO THE RIGHT."
  # "This is the vi for controlling the 6220/6221 current source with a 2182/2182A nanovoltmeter for making delta, diff con, and pulsed IV measurements. You may adapt this code to your needs, but be aware that changes may produce\ninaccurate results or stop the vi from running entirely. For questions regarding this software or for information on how to program the Model 6220/6221 call 1-888-KEITHLEY."
  # "ENABLE BUTTONS AND CONTROLS \nSINCE INITIALIZATION IS NEARLY\nCOMPLETE."
  # "SETUP STEP SOURCE OPTIONS, LOAD DEFAULT IMAGES, LOAD\nDEFAULT INSTRUMENT SETUP, SET FILE OPEN TO TRUE, SET VARS \nFOR FIRST TEST FILE OPEN PROCEDURE."
  # "REGISTRATION, HELP TIPS, \nLOAD DEFAULT PATH, AND \nSCPI COMM ARRAY LOAD."
  # "RESET BUTTONS, INITIALIZE CONTROLS, SET VARS,\nDISABLE SOME CONTROLS DURING STARTUP PROC."
  n1 = flat-sequence {
    tunnel: [w17] -> w1
    tunnel: w1 -> [w43]
    frame #0 {
      w2 = u8 2 ("Disabled")
      w8 = dbl[][] []
      w7 = i32[] [0] ("Complete Waveform")
      w10 = string[] []
      w11 = 0
      w12 = 2
      w3 = TRUE
      w9 = FALSE
      w16 = 2 ("Numeric 2")
      n2 = invoke on="Delta Mode Resistance Graph" class="XYGraph (strict)" method="Reinit To Default"() -> ()  [unwired: 3 in, 3 out]
      n3 = invoke on="Differential Conductance Surface Plot" class="AXCont" method="Reinit To Default"() -> ()  [unwired: 3 in, 3 out]
      n4 = property on="NEW INSTR SETUP" class="Bool"("Disabled"=w16) -> ()  [unwired: 2 in, 2 out]
      n5 = property on="SAVE 2" class="Bool"("Disabled"=w16) -> ()  [unwired: 2 in, 2 out]
      n6 = property on="OPEN" class="Bool (strict)"("Disabled"=w16) -> ()  [unwired: 2 in, 2 out]
      n7 = property on="WEB UPDATES" class="Bool (strict)"("Disabled"=w16) -> ()  [unwired: 2 in, 2 out]
      n8 = property on="GENERATE SCPI - ADVANCED" class="Bool"("Disabled"=w16) -> ()  [unwired: 2 in, 2 out]
      n9 = property on="ABORT DELTA" class="Bool (strict)"("Disabled"=w12) -> ()  [unwired: 2 in, 2 out]
      n10 = property on="RUN DIFF COND" class="Bool"("Disabled"=w11) -> ()  [unwired: 2 in, 2 out]
      n11 = property on="EXIT 2" class="Bool (strict)"("Disabled"=w16) -> ()  [unwired: 2 in, 2 out]
      n12 = property on="ABORT PULSE" class="Bool (strict)"("Disabled"=w12) -> ()  [unwired: 2 in, 2 out]
      n13 = property on="ABORT DIFF COND" class="Bool (strict)"("Disabled"=w12) -> ()  [unwired: 2 in, 2 out]
      n14 = property on="RUN DELTA" class="Bool"("Disabled"=w11) -> ()  [unwired: 2 in, 2 out]
      n15 = property on="RUN PULSE" class="Bool"("Disabled"=w11) -> ()  [unwired: 2 in, 2 out]
      n16 = invoke on="Waveform\n Preview" class="WaveformGraph (strict)" method="Reinit To Default"() -> ()  [unwired: 3 in, 3 out]
      n17 = property on="Advanced Operation Tab" class="TabCtl (strict)"("Value"=T4."Delta Mode Measurements" ("Main Window Tabs")) -> ()  [unwired: 2 in, 2 out]
      n18 = invoke on="Differential Conductance Graph" class="XYGraph (strict)" method="Reinit To Default"() -> ()  [unwired: 3 in, 3 out]
      n19 = property on="Differential Conductance Surface Plot" class="AXCont"("Visible"=TRUE) -> ()  [unwired: 2 in, 2 out]
      n20 = property on="Advanced Operation Tab" class="TabCtl (strict)"("Page Selector Visible"=w3, "Disabled"=w2) -> ()  [unwired: 2 in, 2 out]
      n21 = property on="ScratchPad" class="LstBox (strict)"("Value"=w7, "Item Names"=w10) -> ()  [unwired: 2 in, 2 out]
      n22 = property on="Complete Waveform" class="LstBox (strict)"("Value"=w7, "Item Names"=w10) -> ()  [unwired: 2 in, 2 out]
      n23 = property on="4 step TABS" class="TabCtl (strict)"("Value"=T3."step 1" ("4 step TABS")) -> ()  [unwired: 2 in, 2 out]
      n24 = property on="demo warning" class="Str"("Visible"=w9) -> ()  [unwired: 2 in, 2 out]
      n25 = property on="debug str" class="Str"("Visible"=w9) -> ()  [unwired: 2 in, 2 out]
      n26 = property on="WEB UPDATE STR" class="Str"("Visible"=w9) -> ()  [unwired: 2 in, 2 out]
      n27 = property on="COMM\nTab Control" class="TabCtl (strict)"("Value"=T2."STARTUP" ("COMM\nTab Control")) -> ()  [unwired: 2 in, 2 out]
      n28 = invoke on="Pulsed IV Graph" class="XYGraph (strict)" method="Reinit To Default"() -> ()  [unwired: 3 in, 3 out]
      n29 = property on="DEMO MODE" class="Bool (strict)"("Value"=w9) -> ()  [unwired: 2 in, 2 out]
      n30 = local write "Main Tabs"(T1."General" ("Big Tabs")) -> ()
      n31 = property on="Main Tabs" class="TabCtl (strict)"("Page Selector Visible"=w3, "Disabled"=w2) -> ()  [unwired: 2 in, 2 out]
      "ScratchPad Array" <- w8
      "Complete Array" <- w8
      "ScratchPad Array Cnt" <- w7
      "Complete Array Cnt" <- w7
      "empty" <- dbl[] array[66001 elements]
    }
    frame #1 {
      n32 = Current VI's Path() -> (path=w20:path)
      n33 = Strip Path(path=w20) -> (stripped path=w25:path)  [unwired: 1 out]
      n34 = Path To String(path=w20) -> (string=w21:string)
      n35 = Search/Split String(string=w21, search string/char (-)=".exe") -> (offset of match=w23:i32)  [unwired: 1 in, 2 out]
      n36 = Greater Than 0?(x=w23) -> (x > 0?=w24:bool)
      n37 = case shown="True" w24 {
        tunnel: w25 -> [w33 w35]
        tunnel: [w33 w34] -> w19
        frame False {
        }
        frame True {
          n38 = Strip Path(path=w35) -> (stripped path=w34:path)  [unwired: 1 out]
        }
      }
      n39 = Build Path(base path=w19, name or relative path="data") -> (appended path=w17:path)
      "Default path" <- w17
      n40 = local read "Settings cluster"() -> (w26:T7)
      n41 = call "Register&Tips.vi"("stripped path"=w17, "Settings cluster"=w26, "mail server"="mail server") -> ("WEB UPDATES"=w27:bool, "Settings cluster 2"=→"Settings cluster":T7, "error out 10"=→"error out 10":errorcluster, "error out 7"=→"error out 7":errorcluster)
      n42 = local write "WEB UPDATES"(w27) -> ()
      n43 = call "LoadScpi.vi"("stripped path"=w17) -> ("GPIB Array"=→"GPIB Array":string[])
    }
    frame #2 {
      w58 = FALSE
      n44 = call "StepPicSetup.vi"("stripped path"=w43) -> ("PULSE DIAGRAM"=→"PULSE DIAGRAM":picture, "PULSE DIAGRAM-SWEEP"=→"PULSE DIAGRAM-SWEEP":picture, "Array 2"=w57:string[], "step 1 pic"=→"step 1 pic":picture, "Boolean"=w55:bool, "step 2 pic"=→"step 2 pic":picture, "Array"=w56:T9, "Main intro bar"=→"Main intro bar":picture, "step 3 pic"=→"step 3 pic":picture, "step 4 pic"=→"step 4 pic":picture, "DELTA DIAGRAM"=→"DELTA DIAGRAM":picture, "TREE DIAGRAM"=→"TREE DIAGRAM":picture, "DIFF COND DIAGRAM"=→"DIFF COND DIAGRAM":picture)  [unwired: 1 in, 1 out]
      n45 = Build Path(base path=w43, name or relative path="defaulttest.cfg" ("file path (dialog if empty)")) -> (appended path=w80:path)
      n46 = local write "PULSE HELP TABS"(enum32{"DIAGRAM 2", "DIAGRAM", "TEXT"}."DIAGRAM" ("PULSE HELP TABS")) -> ()
      n47 = control-ref of="CAP IN"() -> (w42:refnum<vi>)
      n48 = call <vilib>:"Read Characters From File.vi"("file path (dialog if empty)"=w80) -> ("character string"=w86:string)  [unwired: 5 in, 3 out]
      n49 = Unflatten From String(type="Default Cluster", binary string=w86) -> (value=w85:T8, error out=w36:errorcluster)  [unwired: 3 in, 1 out]
      n50 = local write "OPEN"(TRUE) -> ()
      n51 = Unbundle(w36) -> ("status"=w82:bool)  [unwired: 2 out]
      n52 = control-ref of="LOW to EARTH 2"() -> (w41:refnum<vi>)
      n53 = control-ref of="DEFAULT setup"() -> (w77:refnum<vi>)
      n54 = control-ref of="Default Cluster"() -> (w76:refnum<vi>)
      n55 = control-ref of="LOW to EARTH"() -> (w70:refnum<vi>)
      n56 = control-ref of="Input instrument IP Address:"() -> (w66:refnum<vi>)
      n57 = control-ref of=".  IP#2"() -> (w65:refnum<vi>)
      n58 = control-ref of=".  IP#3"() -> (w64:refnum<vi>)
      n59 = control-ref of=".  IP#4"() -> (w63:refnum<vi>)
      n60 = control-ref of="Select Network Card number:\n(default to zero)"() -> (w62:refnum<vi>)
      n61 = control-ref of="Select GPIB Address number \nof the current source:"() -> (w61:refnum<vi>)
      n62 = control-ref of="GPIB 6220 label"() -> (w69:refnum<vi>)
      n63 = control-ref of="Select GPIB Board number:\n(default to zero)"() -> (w60:refnum<vi>)
      n64 = control-ref of="Select the current source model number:"() -> (w75:refnum<vi>)
      n65 = control-ref of="Select the nanovoltmeter model number:"() -> (w74:refnum<vi>)
      n66 = control-ref of="The current source is set up for easy cabling in STANDARD CONNECTIONS mode. This \nallows for many versatile measurement setups. However, with high impedance\ndevices or with significant cable capacitance the RC product in the circuit can impact the \ninstrument's risetime for some tests. If you would like to make GUARDED CONNECTIONS\nbecause of the RC present in your test system or for any other reason select GUARDED\nCONNECTIONS below, otherwise use STANDARD CONNECTIONS."() -> (w73:refnum<vi>)
      n67 = control-ref of="Power:"() -> (w71:refnum<vi>)
      n68 = control-ref of="Model 6220 or 6221 is connected by:"() -> (w68:refnum<vi>)
      n69 = control-ref of="Select the interface for the 6220/6221:"() -> (w67:refnum<vi>)
      n70 = control-ref of="HI IMP devices?"() -> (w72:refnum<vi>)
      n71 = case shown="False" w55 {
        tunnel: w57 -> [w89 _]
        tunnel: w56 -> [w88 _]
        frame False {
          n72 = property on="Select step source:" class="Ring (strict)"("Strings []"=w89) -> ()  [unwired: 2 in, 2 out]
          "MASTER DRIVER Array" <- w88
        }
        frame True {
        }
      }
      n73 = property on="Current Test File:" class="Path"("Value"=path "") -> ()  [unwired: 2 in, 2 out]
      n74 = local write "TAKE CONTROL"(FALSE ("TAKE CONTROL")) -> ()
      n75 = property on="OK" class="Bool (strict)"("Disabled"=0) -> ()  [unwired: 2 in, 2 out]
      n76 = call "DefaultSetup.vi"("Default Cluster 3"=w76, "GPIB only Label"=w69, "interface ring"=w67, "IP num 1"=w66, "standard conn"=w73, "IPnum2"=w65, "HiImp conn"=w72, "nV model#"=w74, "Default Cluster 2"=w85, "IP num3"=w64, "Default Cluster"="Default Cluster", "Make default"=w77, "Conn by RING"=w68, "NIC#"=w62, "ISrc model #"=w75, "Lo2 Earth"=w70, "err"=w82, "C IN"=w42, "LO EARTh"=w41, "Power Freq."=w71, "GPIB ADDR#"=w61, "GPIB board#"=w60, "IP num 4"=w63) -> ("Last setup Cluster"=→"Last setup Cluster":T11)  [unwired: 4 in]
      n77 = local write "last amp"("" ("llast amp")) -> ()
      n78 = local write "init"(TRUE ("init")) -> ()
      "EXIT NOW" <- w58
      "SAVE NOW" <- w58
      "STEP EDIT VAR" <- w58
      "FIRST OPEN" <- TRUE
      "UPLOAD TIME WINDOW" <- "            ARB WAVEFORM DATA UPLOAD\n\n\nDepending on the size of the complete waveform it may take a few moments to upload the data. When this window disappears, you may continue by running the waveform. The waveform will be saved in ARB1 and stored in nonvolatile memory. \n"
    }
    frame #3 {
      w105 = 2.0 ("y")
      w91 = u8 66 ("Disabled")
      w115 = FALSE ("Visible")
      w122 = u8 0 ("Disabled")
      w124 = FALSE ("Scalar?")
